vi "ReadEEPROMtoVerify.vi"(8 "error in (no error)":errorcluster, 10 "reference":refnum<k7>, 11 "IN":T1={"step name 1"="", "updata 2"="1000", "limitdata 3"="", "load vi name 4"="", "parameter 5"=""}) -> (0 "error out":errorcluster, 2 "reference out":refnum<k7>, 3 "Cluster":T2)   [LabVIEW 2013]
panel:
  out "error out 2":errorcluster
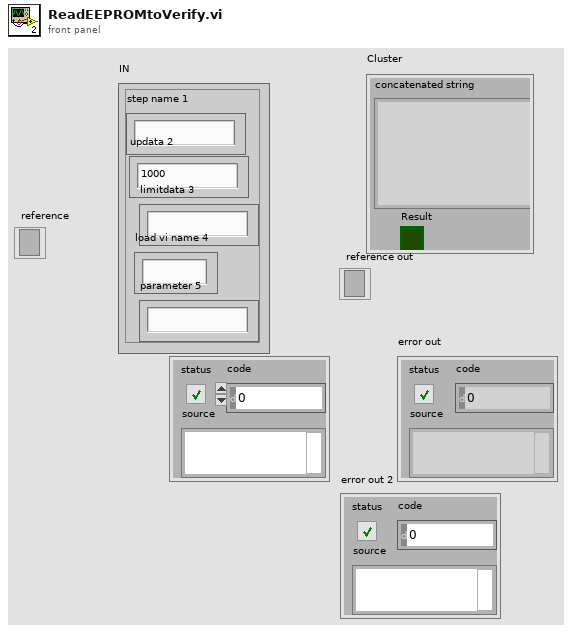
[diagram p1: front panel]
types:
  T1 = cluster{"step name 1":string, "updata 2":string, "limitdata 3":string, "load vi name 4":string, "parameter 5":string}
  T2 = cluster{"concatenated string":string, "Result":bool}
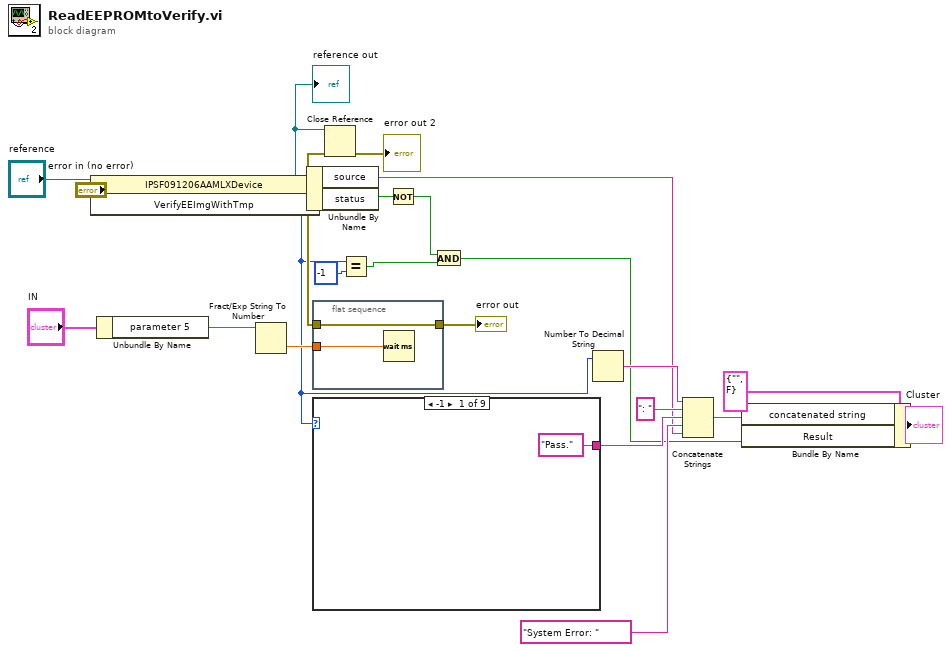
[diagram p0: block diagram]
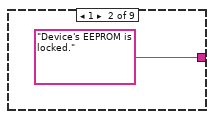
[diagram p2: hidden frame]
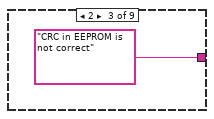
[diagram p3: hidden frame]
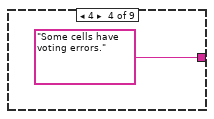
[diagram p4: hidden frame]
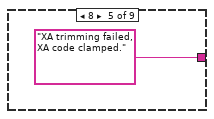
[diagram p5: hidden frame]
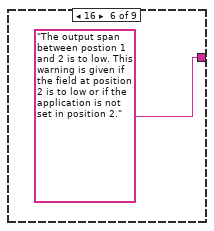
[diagram p6: hidden frame]
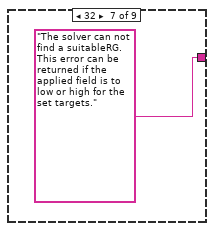
[diagram p7: hidden frame]
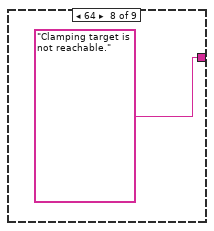
[diagram p8: hidden frame]
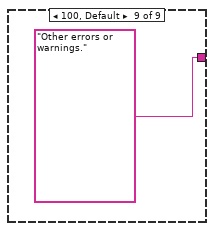
[diagram p9: hidden frame]
diagram:
  n1 = invoke class="IPSF091206AAMLXDevice" method="VerifyEEImgWithTmp"(reference="reference", error in="error in (no error)") -> (reference out=w9:refnum<k7>, error out=w7:errorcluster, "VerifyEEImgWithTmp"=w4:i32)  [unwired: 1 in]
  "reference out" <- w9
  n2 = Unbundle By Name("IN") -> ("parameter 5"=w19:string)
  n3 = Fract/Exp String To Number(string=w19) -> (number=w20:dbl)  [unwired: 3 in, 1 out]
  n4 = Unbundle By Name(w7) -> ("source"=w11:string, "status"=w17:bool)
  n5 = flat-sequence {
    tunnel: w20 -> [w25]
    tunnel: w7 -> [w24]
    tunnel: [w24] -> w8
    frame #0 {
      n6 = Wait (ms)(milliseconds to wait=w25) -> ()  [unwired: 1 out]
    }
  }
  n7 = case shown="-1" w4 {
    tunnel: ["Pass." "Device's EEPROM is locked." "CRC in EEPROM is not correct" "Some cells have voting errors." "XA trimming failed, XA code clamped." "The output span between postion 1 and 2 is to low. This warning is given if the field at position 2 is to low or if the application is not set in position 2." "The solver can not find a suitableRG. This error can be returned if the applied field is to low or high for the set targets." "Clamping target is not reachable." "Other errors or warnings."] -> w13
    frame -1 {
    }
    frame 1 {
    }
    frame 2 {
    }
    frame 4 {
    }
    frame 8 {
    }
    frame 16 {
    }
    frame 32 {
    }
    frame 64 {
    }
    frame 100, Default {
    }
  }
  n8 = Close Reference(reference=w9, error in (no error)=w7) -> (error out=→"error out 2":errorcluster)
  n9 = Equal?(x=w4, y=-1) -> (x = y?=w1:bool)
  n10 = Not(x=w17) -> (.not. x?=w16:bool)
  n11 = And(x=w16, y=w1) -> (x .and. y?=w2:bool)
  n12 = Number To Decimal String(number=w4) -> (decimal integer string=w15:string)  [unwired: 1 in]
  n13 = Concatenate Strings(w15, ": " ("string"), w13, "System Error: " ("string"), w11) -> (w10:string)
  n14 = Bundle By Name(cluster=T2 {"concatenated string"="", "Result"=FALSE} ("Cluster"), "concatenated string"=w10, "Result"=w2) -> (→"Cluster":T2)
  "error out" <- w8
